vi "SIM_CurrentOutput.vi"(9 "array":dbl[][](array[numeric]), 10 "Position (Reframed)":cluster{"x (m)":dbl, "y (m)":dbl, "z (mm)":dbl} {"z (mm)" format="%.1f"; "y (m)" format="%.1p"; "x (m)" format="%.1p"}) -> (3 "Current Out (A)":dbl, 4 "Zread":dbl)   [LabVIEW 2021]
uses:
  <vilib>/ptbypt/NI_PtbyPt.lvlib
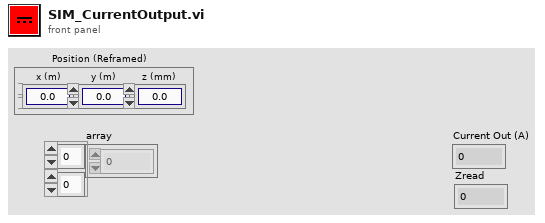
[diagram p1: front panel]
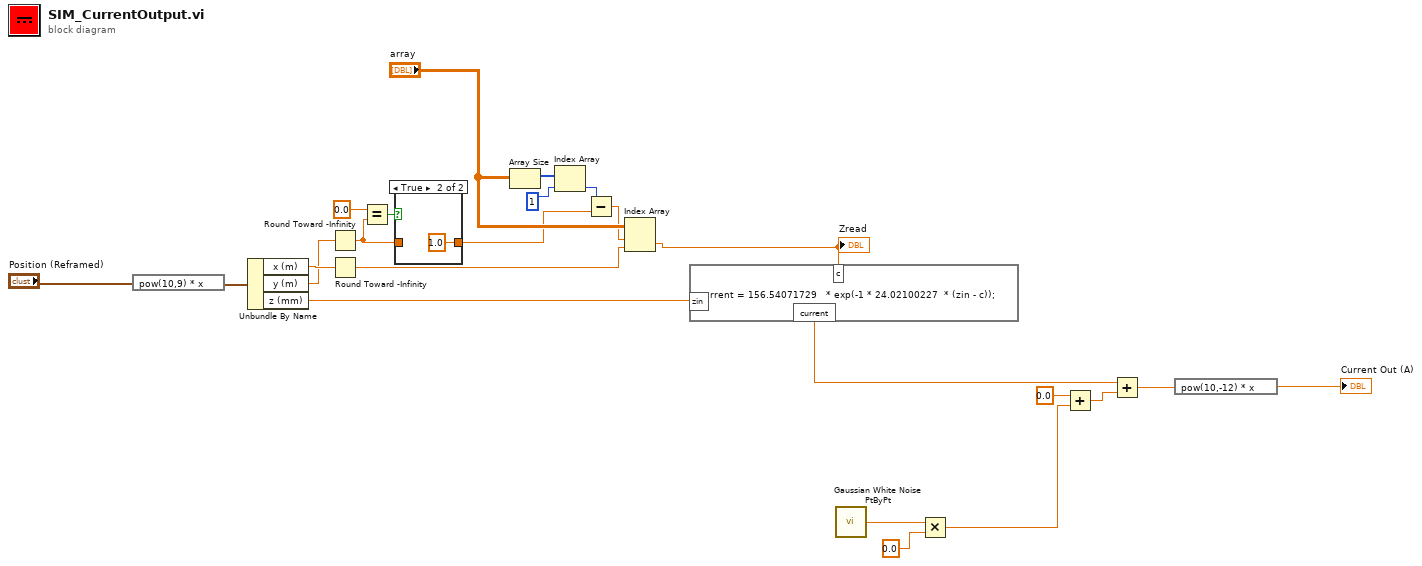
[diagram p0: block diagram]
diagram:
  n1 = expression code="pow(10,9) * x"("Position (Reframed)") -> (w15:cluster{"x (m)":dbl, "y (m)":dbl, "z (mm)":dbl})
  n2 = Unbundle By Name(w15) -> ("x (m)"=w14:dbl, "y (m)"=w13:dbl, "z (mm)"=w12:dbl)
  n3 = Round Toward -Infinity(1:w13) -> (0:w1:dbl)
  n4 = Round Toward -Infinity(1:w14) -> (0:w24:dbl)
  n5 = Equal?(x=0.0, y=w1) -> (x = y?=w4:bool)
  n6 = case shown="True" w4 {
    tunnel: [w25 1.0] -> w2
    tunnel: w1 -> [w25 _]
    frame False {
    }
    frame True {
    }
  }
  n7 = Array Size(array="array") -> (size(s)=w8:i32[])
  n8 = Index Array(array=w8, index=1) -> (element=w5:i32)
  n9 = Subtract(x=w5, y=w2) -> (x-y=w6:dbl)
  n10 = Index Array(array="array", index (row)=w6, index (col)=w24) -> (element=w17:dbl)
  "Zread" <- w17
  n11 = formula code="current = 156.54071729   * exp(-1 * 24.02100227  * (zin - c));"("zin"=w12, "c"=w17) -> ("current"=w18:dbl)
  n12 = call <vilib>:"Gaussian White Noise PtByPt.vi"() -> ("Gaussian white noise"=w23:dbl)  [unwired: 3 in]
  n13 = Multiply(x=w23, y=0.0) -> (x*y=w20:dbl)
  n14 = Add(x=0.0, y=w20) -> (x+y=w21:dbl)
  n15 = Add(x=w18, y=w21) -> (x+y=w11:dbl)
  n16 = expression code="pow(10,-12) * x"(w11) -> (→"Current Out (A)":dbl)
